vi "ApplySwitchExecConfigurationFile.vi"(7 "Virtual Device Name":string, 8 "error in (no error)":errorcluster, 11 "SwitchExec Configuration File (*.txt)":path) -> (0 "error out":errorcluster)   [LabVIEW 2009]
panel:
  # "Applying Switch Configuration"
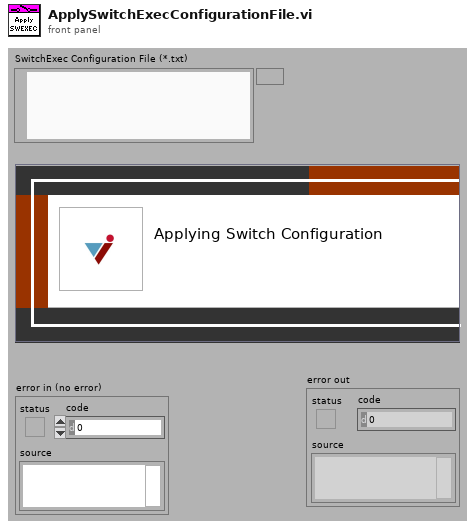
[diagram p1: front panel]
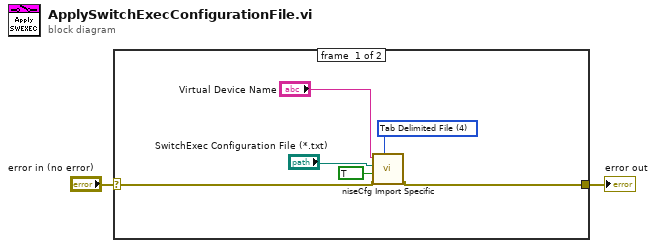
[diagram p0: block diagram]
diagram:
  n1 = case shown="No Error" "error in (no error)" {
    selector: "error in (no error)" -> [w8 w9]
    tunnel: [w7 w9] -> w1
    frame #0 {
      w3 = 4 items=["NI Switch Executive Export File"=1, "Excel XLS Workbook"=2, "Excel XLSX Workbook"=3, "Tab Delimited File"=4] ("File Format")
      n2 = call <vilib>:"niseCfg Import Specific.vi"("File Format"=w3, "error in (no error)"=w8, "Overwrite Existing (False)"=TRUE, "Path"="SwitchExec Configuration File (*.txt)", "Virtual Device Name"="Virtual Device Name") -> ("error out"=w7:errorcluster)  [unwired: 6 in]
    }
    frame #1 {
    }
  }
  "error out" <- w1
